vi "Convert_Result_Num_Boolean.vi"(4 "Number_Result":u16) -> (1 "Boolean_Result":bool=TRUE)   [LabVIEW 2017]
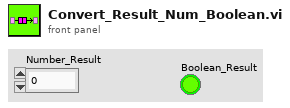
[diagram p1: front panel]
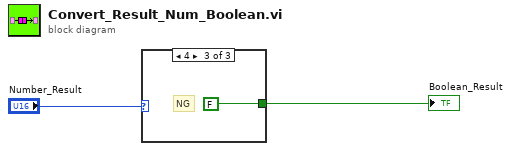
[diagram p0: block diagram]
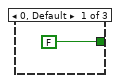
[diagram p2: hidden frame]
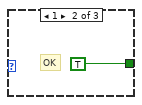
[diagram p3: hidden frame]
diagram:
  n1 = case shown="4" "Number_Result" {
    tunnel: [FALSE TRUE FALSE] -> w1
    frame 0, Default {
    }
    frame 1 {
      # "OK"
    }
    frame 4 {
      # "NG"
    }
  }
  "Boolean_Result" <- w1
